vi "sql time log.vi"() -> ()   [LabVIEW 2017]
uses:
  <vilib>/addons/database/Connection.llb/DB Tools Open Connec (Path).vi
  <vilib>/addons/database/Connection.llb/Conn Execute.vi
  <vilib>/addons/database/Recordset.llb/Rec Fetch Recordset Data (R).vi
  <vilib>/addons/database/Recordset.llb/Rec Destroy - Connection.vi
  <vilib>/addons/database/NI_Database_API.lvlib
panel:
  in  "stop":bool
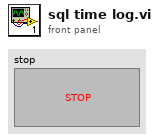
[diagram p1: front panel]
types:
  T1 = typedef "NI_Database_API.lvlib/Conn ObjectReference.ctl" = refnum<k1>
  T2 = typedef "NI_Database_API.lvlib/Rec ObjectReference.ctl" = refnum<k1>
  T3 = cluster{i32, "seconds since 1Jan1904":timestamp, "date/time string":string, "standard output":string, i32}
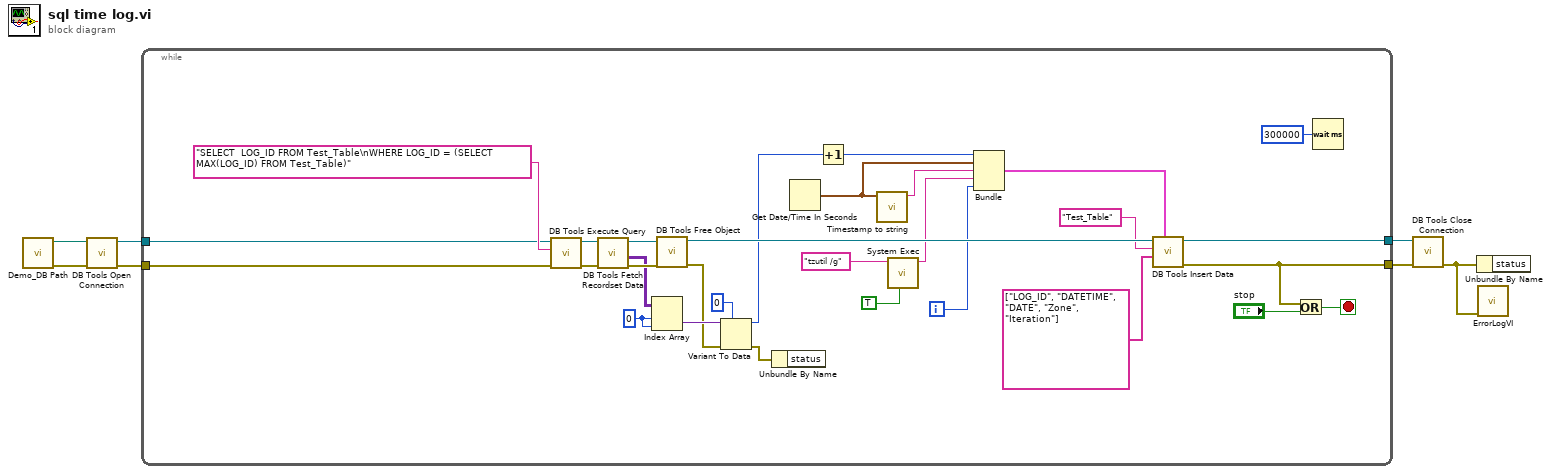
[diagram p0: block diagram]
diagram:
  n1 = call "Demo_DB Path.vi"() -> ("error out"=w6:errorcluster, "DB Path"=w7:path)  [unwired: 10 in]
  n2 = call-poly <vilib>:"DB Tools Open Connection.vi"("error in (no error)"=w6, "connection information"=w7) -> ("error out"=w5:errorcluster, "connection reference"=w4:T1)  [unwired: 6 in]
  n3 = while {
    tunnel: w5 -> [w27]
    tunnel: w4 -> [w26]
    tunnel: [w21] -> w3
    tunnel: [w20] -> w2
    i -> [w11]
    stop <- w18 stop-if-true
    w30 = 0 ("index (row)")
    n4 = call-poly <vilib>:"DB Tools Execute Query.vi"("error in (no error)"=w27, "SQL query"="SELECT  LOG_ID FROM Test_Table\nWHERE LOG_ID = (SELECT MAX(LOG_ID) FROM Test_Table)", "connection reference"=w26) -> ("error out"=w32:errorcluster, "recordset reference"=w31:T2)  [unwired: 5 in]
    n5 = call-poly <vilib>:"DB Tools Fetch Recordset Data.vi"("error in (no error)"=w32, "recordset reference"=w31) -> ("error out"=w35:errorcluster, "recordset data"=w34:variant[][], "recordset reference out"=w36:T2)  [unwired: 3 in]
    n6 = Index Array(array=w34, index (row)=w30, index (col)=w30) -> (element=w37:variant)
    n7 = call-poly <vilib>:"DB Tools Free Object.vi"("error in (no error)"=w35, "recordset reference"=w36) -> ("error out"=w33:errorcluster, "connection reference"=w24:T1)  [unwired: 8 in]
    n8 = Variant To Data(error in=w33, type=0, Variant=w37) -> (data=w23:i32, error out=w15:errorcluster)
    n9 = Unbundle By Name(w15) -> ()  [unwired: 1 out]
    n10 = Get Date/Time In Seconds() -> (seconds since 1Jan1904=w8:timestamp)
    n11 = Increment(x=w23) -> (x+1=w9:i32)
    n12 = call "Timestamp to string.vi"("time stamp"=w8) -> ("date/time string"=w22:string)  [unwired: 8 in, 2 out]
    n13 = call <vilib>:"System Exec.vi"("run minimized? (F)"=TRUE, "command line"="tzutil /g") -> ("standard output"=w12:string)  [unwired: 6 in, 3 out]
    n14 = Bundle(w9, "seconds since 1Jan1904"=w8, "date/time string"=w22, "standard output"=w12, w11) -> (w25:T3)  [unwired: 1 in]
    n15 = call <vilib>:"DB Tools Insert Data.vi"("data"=w25, "columns"=string[] ["LOG_ID", "DATETIME", "DATE", "Zone", "Iteration"], "table"="Test_Table", "connection reference"=w24) -> ("error out"=w20:errorcluster, "connection reference out"=w21:T1)  [unwired: 6 in]
    n16 = Or(x=w20, y="stop") -> (x .or. y?=w18:bool)
    n17 = Wait (ms)(milliseconds to wait=u32 300000) -> ()  [unwired: 1 out]
  }
  n18 = call <vilib>:"DB Tools Close Connection.vi"("error in (no error)"=w2, "connection reference"=w3) -> ("error out"=w1:errorcluster)  [unwired: 5 in]
  n19 = Unbundle By Name(w1) -> ()  [unwired: 1 out]
  n20 = call "ErrorLogVI.vi"("Error In"=w1) -> ()  [unwired: 11 in]
